vi "io_clear_before_read.vi"(6 "Block Logging (F)":bool, 8 "error in":errorcluster, 11 "VISA resource name":refnum<visa-resource-name>) -> (0 "error out":errorcluster, 3 "VISA resource name out":refnum<visa-resource-name>)   [LabVIEW 2014, in "rszvl_rsidr_core.lvlib"]
uses:
  rszvl_rsidr_core.lvlib
  type_Error_Codes.ctl
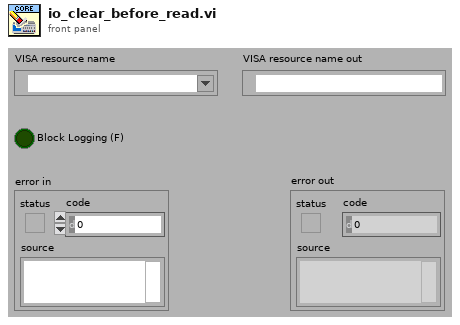
[diagram p1: front panel]
types:
  T1 = typedef "rszvl_rsidr_core.lvlib/type_Error_Codes.ctl" = enum16{"No_error", "VISA_err_ResourceNotFound", "VISA_err_Timeout", "VISA_warn_MoreDataAvailable", "RS_err_MissingCallback", "RS_err_InvalidAttribute", "RS_err_InvalidValue", "RS_err_UnknownResource", "RS_err_AlreadyInitialized", "RS_err_InstrumentStatus", "RS_err_BadRepCapName", "RS_err_TypesMismatch", "RS_err_ValueNotSupported", "RS_err_InvalidRngTable", "RS_err_IDqueryFail", "RS_err_UnexpResponse", "VISA_warn_ConfigNotLoaded", "RS_err_AttributeNotReadable", "RS_err_AttributeNotWritable", "RS_err_InstrumentType", "RS_err_InstrumentOption", "VISA_err_InvalidSize", "RS_err_ReliabilityIndicator", "VISA_warn_UnknownStatus", "VISA_warn_TermCharRead", "VISA_err_IO_error"}
  T2 = typedef "rszvl_rsidr_core.lvlib/type_Session_Data.ctl" = cluster{"Instr type":string, "Instr type for err. msg.":string, "Installed Options":string[], "OPC Timeout":i32, "Query Instrument Status":bool, "Check Range":bool, "Check Options":bool, "Add LF to Write":bool, "Simulate":bool, "Logging":bool, "Logging params":variant, "Interface Type":enum16{"Unknown", "GPIB", "VXI", "GPIB_VXI", "ASRL", "PXI", "TCPIP", "USB", "SOCKET"}, "Fast Sweep":i32, "AdditionalFlags":i32, "WaitBeforeWrite":i32, "WaitBeforeRead":i32, "BinDataChunkSize":i64}
  T3 = enum16{"Unknown", "GPIB", "VXI", "GPIB_VXI", "ASRL", "PXI", "TCPIP", "USB", "SOCKET"}
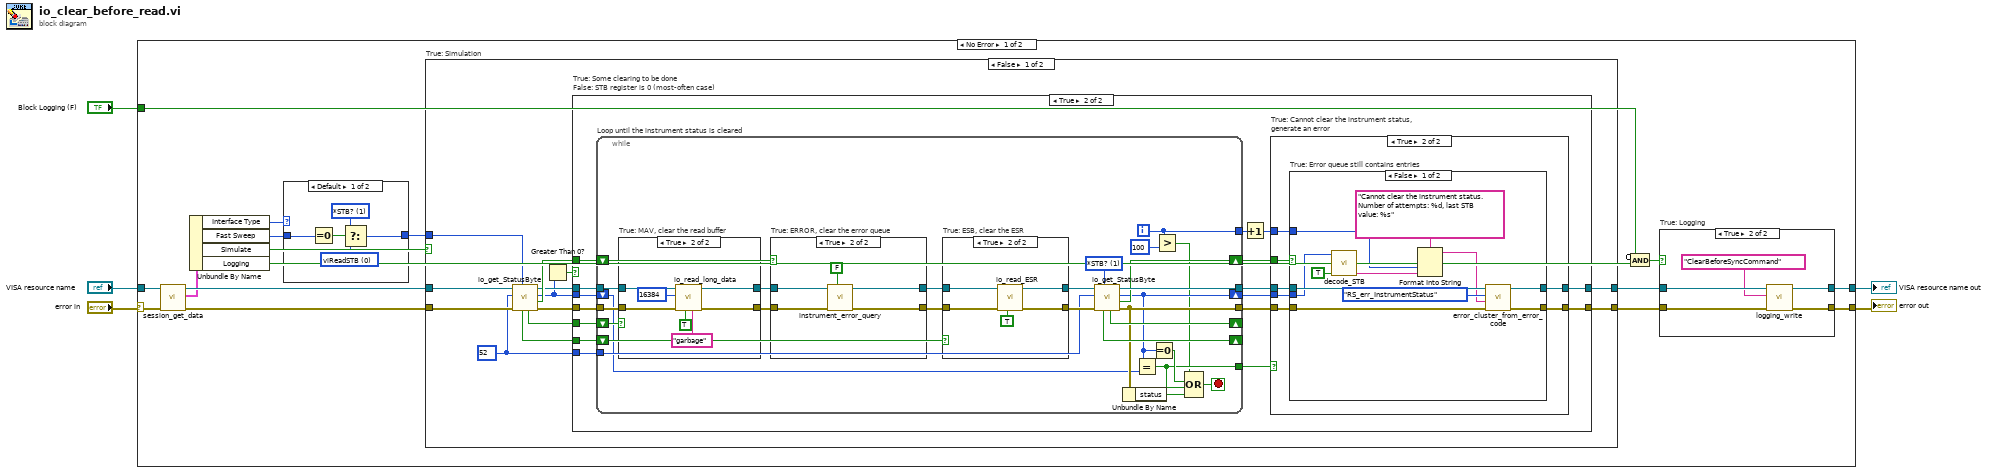
[diagram p0: block diagram]
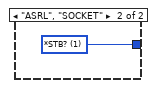
[diagram p2: hidden frame]
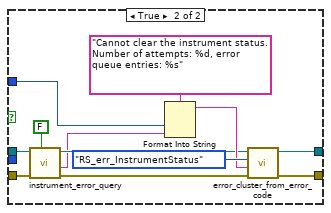
[diagram p6: hidden frame]
diagram:
  n1 = case shown="No Error" "error in" {
    selector: "error in" -> [w21 w151]
    tunnel: [w15 w151] -> w5
    tunnel: "VISA resource name" -> [w20 w150]
    tunnel: [w12 w150] -> w2
    tunnel: "Block Logging (F)" -> [w9 _]
    frame No Error {
      n2 = call "session_get_data.vi"("error in"=w21, "VISA resource name"=w20) -> ("error out"=w19:errorcluster, "Session User Data out"=w17:T2, "VISA resource name out"=w18:refnum<visa-resource-name>)  [unwired: 7 in]
      n3 = Unbundle By Name(w17) -> ("Interface Type"=w8:T3, "Fast Sweep"=w7:i32, "Simulate"=w16:bool, "Logging"=w11:bool)
      n4 = case shown="Default" w8 {
        tunnel: w7 -> [w23 _]
        tunnel: [w22 w27] -> w6
        frame Default {
          w26 = u16 0 items=["viReadSTB", "*STB?"] ("Method (viReadSTB)")
          w25 = u16 1 items=["viReadSTB", "*STB?"] ("Method (viReadSTB)")
          n5 = Equal To 0?(x=w23) -> (x = 0?=w24:bool)
          n6 = Select(t=w25, s=w24, f=w26) -> (s? t:f=w22:u16)
        }
        frame "ASRL", "SOCKET" {
          w27 = u16 1 items=["viReadSTB", "*STB?"] ("Method (viReadSTB)")
        }
      }
      n7 = case "True: Simulation" shown="False" w16 {
        tunnel: [w39 w149] -> w14
        tunnel: w19 -> [w47 w149]
        tunnel: w18 -> [w46 w148]
        tunnel: [w38 w148] -> w13
        tunnel: w6 -> [w35 _]
        frame False {
          w37 = u16 52 ("y")
          n8 = call "io_get_StatusByte.vi"("Method (viReadSTB)"=w35, "error in"=w47, "Bits filter (None - 0xFF)"=w37, "VISA resource name"=w46) -> ("error out"=w41:errorcluster, "Error"=w43:bool, "STB returned"=w36:u16, "VISA resource name out"=w40:refnum<visa-resource-name>, "MAV"=w42:bool, "OPC (ESB)"=w45:bool)  [unwired: 2 in]
          n9 = Greater Than 0?(x=w36) -> (x > 0?=w44:bool)
          n10 = case "True: Some clearing to be done\nFalse: STB register is 0 (most-often case)" shown="True" w44 {
            tunnel: w41 -> [w49 w62]
            tunnel: w45 -> [_ w65]
            tunnel: w43 -> [_ w64]
            tunnel: w42 -> [_ w63]
            tunnel: w40 -> [w48 w61]
            tunnel: [w49 w56] -> w39
            tunnel: [w48 w55] -> w38
            tunnel: w37 -> [_ w60]
            tunnel: w36 -> [_ w59]
            frame False {
            }
            frame True {
              n11 = while "Loop until the instrument status is cleared" {
                tunnel: w62 -> [w122]
                shift-right: [w109] -> _
                shift-left: w65 -> [w118]
                shift-right: [w111] -> w52
                shift-left: w64 -> [w123]
                shift-right: [w110] -> _
                shift-left: w63 -> [w124]
                tunnel: w61 -> [w121]
                tunnel: [w107] -> w58
                tunnel: [w113] -> w57
                tunnel: w60 -> [w108]
                shift-right: [w105] -> w53
                shift-left: w59 -> [w106]
                tunnel: [w103] -> w54
                tunnel: [w98] -> w51
                i -> [w98]
                stop <- w101 stop-if-true
                w112 = u16 1 items=["viReadSTB", "*STB?"] ("Method (viReadSTB)")
                n12 = case "True: MAV, clear the read buffer" shown="True" w124 {
                  tunnel: w122 -> [w140 w144]
                  tunnel: w121 -> [w139 w143]
                  tunnel: [w140 w142] -> w120
                  tunnel: [w139 w141] -> w119
                  frame False {
                  }
                  frame True {
                    n13 = call "io_read_long_data.vi"("Simulation read buffer (\"Simulation\")"="garbage" ("Simulation read buffer \n(\"Simulation\")"), "Block Logging (F)"=TRUE, "error in"=w144, "Max chunk read bytes count (65536)"=u32 16384, "VISA resource name"=w143) -> ("error out"=w142:errorcluster, "VISA resource name out"=w141:refnum<visa-resource-name>)  [unwired: 3 in, 2 out]
                  }
                }
                n14 = case "True: ERROR, clear the error queue" shown="True" w123 {
                  tunnel: w120 -> [w133 w137]
                  tunnel: w119 -> [w132 w138]
                  tunnel: [w133 w135] -> w117
                  tunnel: [w132 w134] -> w116
                  frame False {
                  }
                  frame True {
                    n15 = call "instrument_error_query.vi"("Add instrument error to error cluster (T)"=FALSE, "error in"=w137, "VISA resource name"=w138) -> ("error out"=w135:errorcluster, "VISA resource name out"=w134:refnum<visa-resource-name>)  [unwired: 5 in, 2 out]
                  }
                }
                n16 = case "True: ESB, clear the ESR" shown="True" w118 {
                  tunnel: w117 -> [w126 w131]
                  tunnel: w116 -> [w125 w130]
                  tunnel: [w126 w129] -> w115
                  tunnel: [w125 w128] -> w114
                  frame False {
                  }
                  frame True {
                    n17 = call "io_read_ESR.vi"("Block Logging (F)"=TRUE, "error in"=w131, "VISA resource name"=w130) -> ("error out"=w129:errorcluster, "VISA resource name out"=w128:refnum<visa-resource-name>)  [unwired: 6 in, 1 out]
                  }
                }
                n18 = call "io_get_StatusByte.vi"("Method (viReadSTB)"=w112, "error in"=w115, "Bits filter (None - 0xFF)"=w108, "VISA resource name"=w114) -> ("error out"=w107:errorcluster, "Error"=w111:bool, "STB returned"=w105:u16, "VISA resource name out"=w113:refnum<visa-resource-name>, "MAV"=w110:bool, "OPC (ESB)"=w109:bool)  [unwired: 2 in]
                n19 = Unbundle By Name(w107) -> ("status"=w102:bool)
                n20 = Equal?(x=w105, y=w106) -> (x = y?=w103:bool)
                n21 = Equal To 0?(x=w105) -> (x = 0?=w104:bool)
                n22 = Greater?(x=w98, y=100) -> (0:w99:bool)
                n23 = Compound Arithmetic op=OR(w99, w104, w103, w102) -> (w101:bool)
              }
              n24 = Increment(x=w51) -> (x+1=w50:i32)
              n25 = case "True: Cannot clear the instrument status,\ngenerate an error" shown="True" w54 {
                tunnel: w58 -> [w67 w74]
                tunnel: w57 -> [w66 w73]
                tunnel: [w67 w72] -> w56
                tunnel: [w66 w71] -> w55
                tunnel: w53 -> [_ w70]
                tunnel: w52 -> [_ w68]
                tunnel: w50 -> [_ w69]
                frame False {
                }
                frame True {
                  n26 = case "True: Error queue still contains entries" shown="False" w68 {
                    tunnel: w74 -> [w85 w90]
                    tunnel: w73 -> [w84 w91]
                    tunnel: [w83 w97] -> w72
                    tunnel: [w82 w96] -> w71
                    tunnel: w70 -> [w78 _]
                    tunnel: w69 -> [w75 w92]
                    frame False {
                      n27 = call "decode_STB.vi"("Compose Summary String  (F)"=TRUE, "STB in"=w78) -> ("Summary string"=w76:string)  [unwired: 6 in, 3 out]
                      n28 = Format Into String(format string="Cannot clear the instrument status. Number of attempts: %d, last STB value: %s" ("error message (\"\")"), w75, w76) -> (resulting string=w79:string)  [unwired: 2 in, 1 out]
                      n29 = call "error_cluster_from_error_code.vi"("error in"=w85, "error message (\"\")"=w79, "Error Enum in"=type_Error_Codes."RS_err_InstrumentStatus", "VISA resource name"=w84) -> ("error out"=w83:errorcluster, "VISA resource name out"=w82:refnum<visa-resource-name>)  [unwired: 6 in]
                    }
                    frame True {
                      n30 = call "instrument_error_query.vi"("Add instrument error to error cluster (T)"=FALSE, "error in"=w90, "VISA resource name"=w91) -> ("error out"=w88:errorcluster, "Error Message(s) out"=w86:string, "VISA resource name out"=w89:refnum<visa-resource-name>)  [unwired: 5 in, 1 out]
                      n31 = Format Into String(format string="Cannot clear the instrument status. Number of attempts: %d, error queue entries: %s" ("error message (\"\")"), w92, w86) -> (resulting string=w93:string)  [unwired: 2 in, 1 out]
                      n32 = call "error_cluster_from_error_code.vi"("error in"=w88, "error message (\"\")"=w93, "Error Enum in"=type_Error_Codes."RS_err_InstrumentStatus", "VISA resource name"=w89) -> ("error out"=w97:errorcluster, "VISA resource name out"=w96:refnum<visa-resource-name>)  [unwired: 6 in]
                    }
                  }
                }
              }
            }
          }
        }
        frame True {
        }
      }
      n33 = Compound Arithmetic op=AND(invert w9, w11) -> (w10:bool)
      n34 = case "True: Logging" shown="True" w10 {
        tunnel: w14 -> [w29 w34]
        tunnel: [w29 w32] -> w15
        tunnel: w13 -> [w28 w33]
        tunnel: [w28 w31] -> w12
        frame False {
        }
        frame True {
          n35 = call "logging_write.vi"("error in"=w34, "String to write"="ClearBeforeSyncCommand", "VISA resource name"=w33) -> ("error out"=w32:errorcluster, "VISA resource name out"=w31:refnum<visa-resource-name>)  [unwired: 7 in]
        }
      }
    }
    frame Error {
    }
  }
  "VISA resource name out" <- w2
  "error out" <- w5
